vi "controlRtOutSignalMode.vi"(7 "Set":bool, 8 "error in":errorcluster, 9 "RT out Mode in":i32, 11 "connection ID":refnum<k5>) -> (0 "error out":errorcluster, 1 "RT out Mode out":i32, 3 "connection ID":refnum<k5>)   [LabVIEW 2016]
panel:
  in  "Set Command":string="com.attocube.amc.rtout.setRtOutSignalMode"
  in  "Get Command":string="com.attocube.amc.rtout.getRtOutSignalMode"
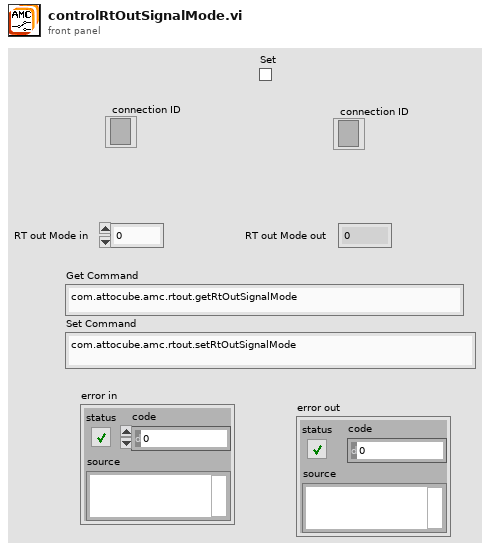
[diagram p1: front panel]
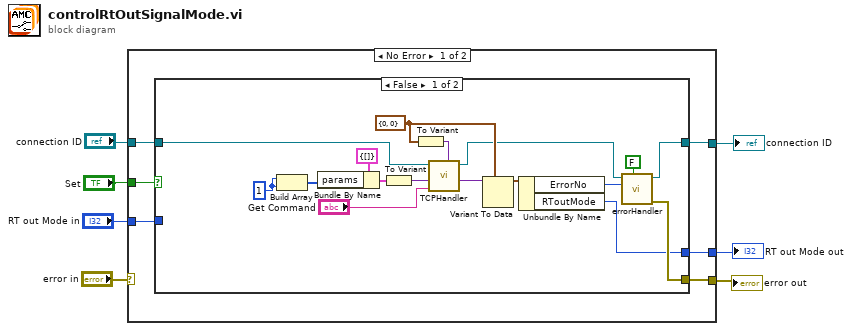
[diagram p0: block diagram]
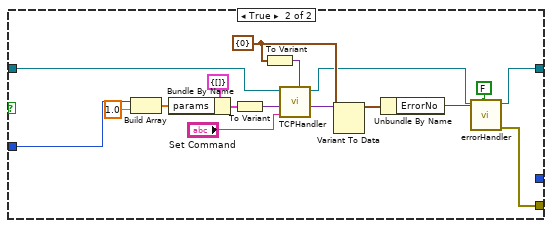
[diagram p2: hidden frame]
diagram:
  n1 = case shown="No Error" "error in" {
    selector: "error in" -> [_ w49]
    tunnel: [w8 w49] -> w7
    tunnel: "Set" -> [w12 _]
    tunnel: [w10 w48] -> w5
    tunnel: "connection ID" -> [w11 w48]
    tunnel: "RT out Mode in" -> [w13 w50]
    tunnel: [w9 w50] -> w2
    frame No Error {
      n2 = case shown="False" w12 {
        tunnel: [w14 w31] -> w10
        tunnel: w11 -> [w21 w42]
        tunnel: [w22 w38] -> w8
        tunnel: [w18 _] -> w9
        tunnel: w13 -> [_ w34]
        frame False {
          w16 = u8 1 ("element")
          w19 = cluster{"ErrorNo":i16, "RToutMode":i64} {"ErrorNo"=0, "RToutMode"=0} ("input cluster")
          n3 = Build Array(w16, w16) -> (w26:u8[])
          n4 = Bundle By Name(cluster=cluster{"params":i16[]} {"params"=[]} ("input cluster"), "params"=w26) -> (w27:cluster{"params":i16[]})
          n5 = To Variant(anything=w27) -> (Variant=w28:variant)
          n6 = To Variant(anything=w19) -> (Variant=w20:variant)
          n7 = call "TCPHandler.vi"("result Types"=w20, "method"="Get Command", "params"=w28, "connection ID"=w21) -> ("result"=w24:variant, "connection ID"=w15:refnum<k5>)  [unwired: 5 in, 1 out]
          n8 = Variant To Data(type=w19, Variant=w24) -> (data=w29:cluster{"ErrorNo":i16, "RToutMode":i64})  [unwired: 1 in, 1 out]
          n9 = Unbundle By Name(w29) -> ("ErrorNo"=w30:i16, "RToutMode"=w18:i64)
          n10 = call "errorHandler.vi"("show popup"=FALSE, "error number"=w30, "connection ID"=w15) -> ("error out"=w22:errorcluster, "connection ID"=w14:refnum<k5>)  [unwired: 7 in]
        }
        frame True {
          w36 = cluster{"ErrorNo":i16} {"ErrorNo"=0} ("input cluster")
          n11 = Build Array(w34, 1.0 ("element")) -> (w44:dbl[])
          n12 = Bundle By Name(cluster=cluster{"params":i64[]} {"params"=[]} ("input cluster"), "params"=w44) -> (w43:cluster{"params":i64[]})
          n13 = To Variant(anything=w43) -> (Variant=w41:variant)
          n14 = To Variant(anything=w36) -> (Variant=w37:variant)
          n15 = call "TCPHandler.vi"("result Types"=w37, "method"="Set Command", "params"=w41, "connection ID"=w42) -> ("result"=w46:variant, "connection ID"=w32:refnum<k5>)  [unwired: 5 in, 1 out]
          n16 = Variant To Data(type=w36, Variant=w46) -> (data=w40:cluster{"ErrorNo":i16})  [unwired: 1 in, 1 out]
          n17 = Unbundle By Name(w40) -> ("ErrorNo"=w39:i16)
          n18 = call "errorHandler.vi"("show popup"=FALSE, "error number"=w39, "connection ID"=w32) -> ("error out"=w38:errorcluster, "connection ID"=w31:refnum<k5>)  [unwired: 7 in]
        }
      }
    }
    frame Error {
    }
  }
  "error out" <- w7
  "connection ID" <- w5
  "RT out Mode out" <- w2
